vi "List Columns.vi"(8 "error in (no error)":errorcluster, 10 "Table name":string, 11 "database in":path) -> (0 "error out":errorcluster, 1 "PRAGMA table info":string[][](array[string]), 2 "Column types":string[](array[string]), 3 "Column names":string[](array[string]))   [LabVIEW 2020, in "sqlite3.lvlib"]
uses:
  sqlite3.lvlib
  sqlite/VIs/open v2.vi
  sqlite/VIs/prepare v2.vi
  sqlite/VIs/step.vi
  sqlite/VIs/column count.vi
  compound/Column.vi
  compound/Resolve Result Type.vi
  sqlite/VIs/finalize.vi
  sqlite/VIs/close v2.vi
  sqlite/subvi/Error Converter (ErrCode or Status).vi
  sqlite/VIs/column text.vi
  sqlite/VIs/column bytes.vi
  sqlite/VIs/column blob.vi
  utilities/MoveBlock.vi
  sqlite/VIs/column type.vi
  sqlite/VIs/errstr.vi
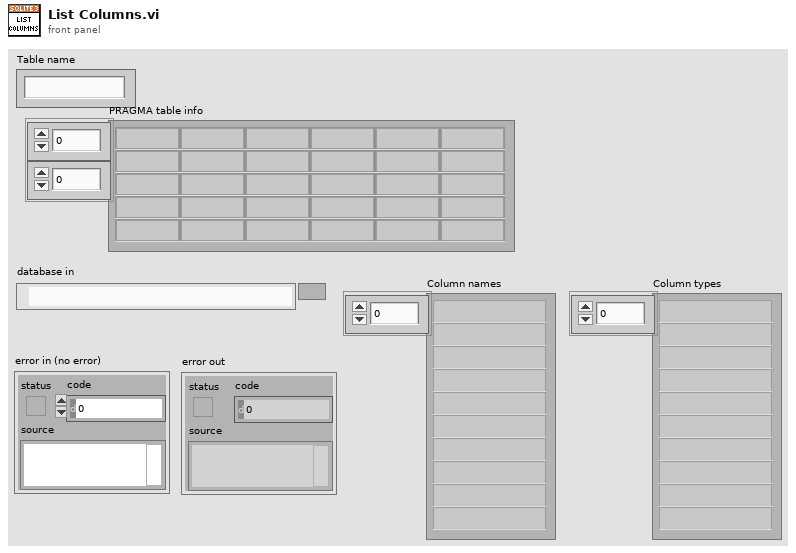
[diagram p1: front panel]
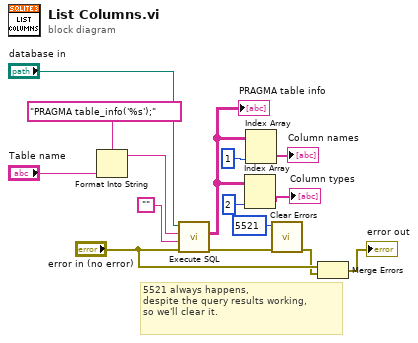
[diagram p0: block diagram]
diagram:
  # "5521 always happens, \ndespite the query results working,\nso we'll clear it."
  n1 = Format Into String(format string="PRAGMA table_info('%s');", "Table name") -> (resulting string=w9:string)  [unwired: 2 in, 1 out]
  n2 = call "Execute SQL.vi"("error in (no error)"="error in (no error)", "[disabled] return type (string)"="", "sql (string)"=w9, "database in"="database in") -> ("error out"=w5:errorcluster, "Query Result"=w8:string[][])  [unwired: 6 in]
  "PRAGMA table info" <- w8
  n3 = Index Array(array=w8, index (col)=2 ("disabled index (col)")) -> (element=→"Column types":string[])  [unwired: 1 in]
  n4 = Index Array(array=w8, index (col)=1 ("index (row)")) -> (element=→"Column names":string[])  [unwired: 1 in]
  n5 = call <vilib>:"Clear Errors.vi"("error in (no error)"=w5, "specific error code to clear (0: all)"=5521) -> ("error out"=w2:errorcluster)  [unwired: 4 in, 1 out]
  n6 = Merge Errors("error in (no error)", w2) -> (→"error out":errorcluster)
